vi "GraphsChartsExperimentation.vi"() -> ()   [LabVIEW 2018]
panel:
  out "Waveform Graph":dbl[](graph)
  out "Waveform Chart":dbl(graph)
  out "Numeric P":dbl
  out "Numeric K":dbl
  in  "Fusão da agua":dbl
  in  "Embulição da agua":dbl
  out "Sua Escala":dbl(slide) scale=-400.0..400.0
  out "Kelvin":dbl(slide) scale=220.0..420.0
  in  "stop":bool
  out "NumericºC":dbl
  out "Numeric ºF":dbl
  out "Temperatura ºC":dbl(slide) scale=-50.0..150.0
  in  "Tempratura (ºF)":dbl(slide) scale=-50.0..300.0
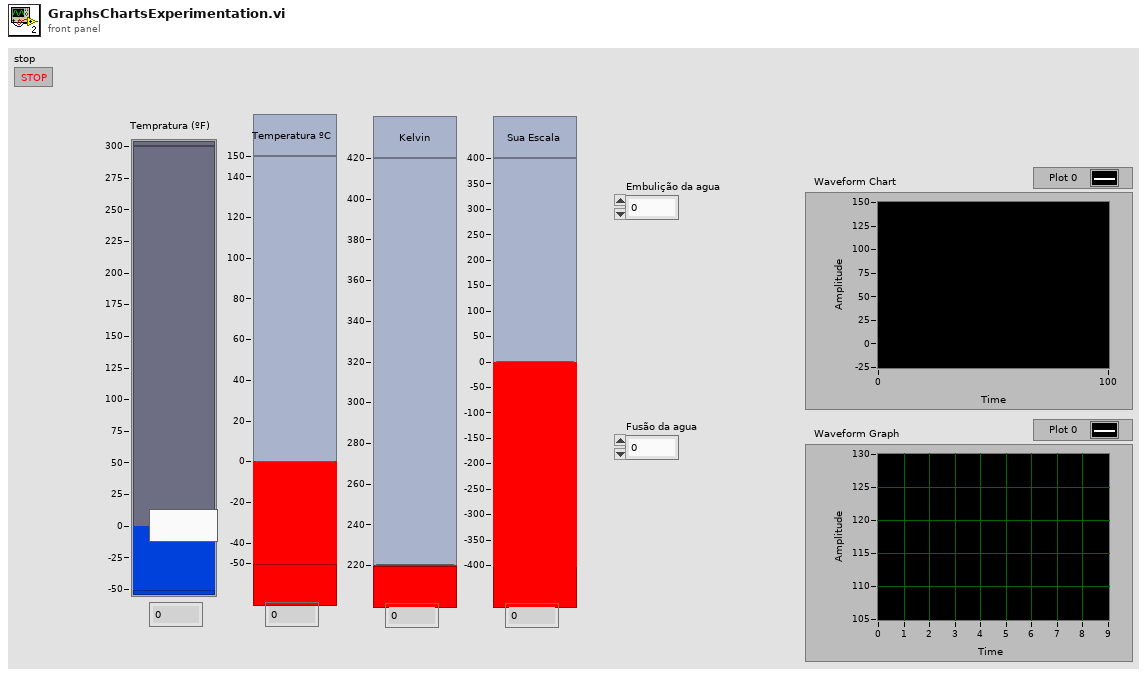
[diagram p1: front panel]
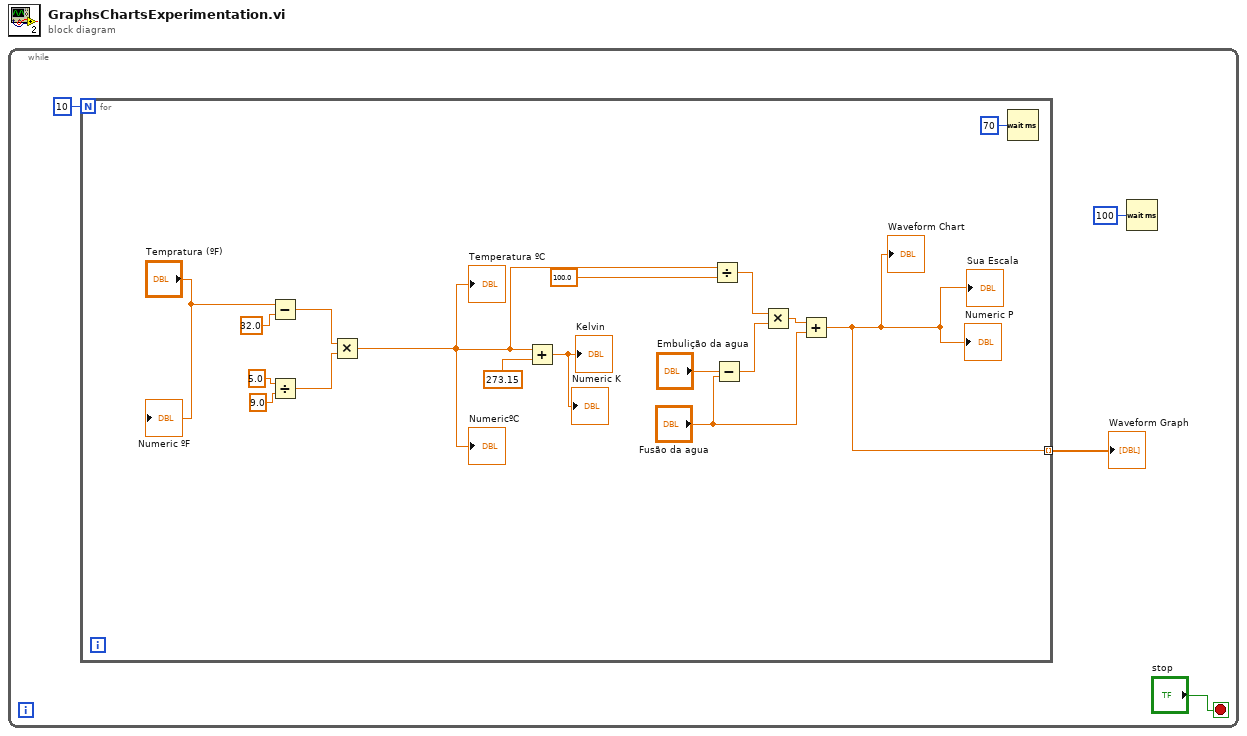
[diagram p0: block diagram]
diagram:
  n1 = while {
    stop <- "stop" stop-if-true
    n2 = for {
      N: 10 -> [_]
      tunnel: [w5] -> w4 mode=indexing
      n3 = Subtract(x="Tempratura (ºF)", y=32.0) -> (x-y=w21:dbl)
      n4 = Divide(x=5.0, y=9.0) -> (x/y=w20:dbl)
      n5 = Multiply(x=w21, y=w20) -> (x*y=w12:dbl)
      "Temperatura ºC" <- w12
      "NumericºC" <- w12
      n6 = Add(x=w12, y=273.15) -> (x+y=→"Kelvin" →"Numeric K":dbl)
      n7 = Divide(x=w12, y=100.0) -> (x/y=w9:dbl)
      n8 = Subtract(x="Embulição da agua", y="Fusão da agua") -> (x-y=w8:dbl)
      n9 = Multiply(x=w9, y=w8) -> (x*y=w7:dbl)
      n10 = Add(x=w7, y="Fusão da agua") -> (x+y=w5:dbl)
      "Sua Escala" <- w5
      "Numeric P" <- w5
      "Waveform Chart" <- w5
      n11 = Wait (ms)(milliseconds to wait=u32 70) -> ()  [unwired: 1 out]
      "Numeric ºF" <- "Tempratura (ºF)"
    }
    "Waveform Graph" <- w4
    n12 = Wait (ms)(milliseconds to wait=u32 100) -> ()  [unwired: 1 out]
  }
